vi "Load Display Settings.vi"(8 "error in (no error)":errorcluster, 11 "AF IMAQ Display in":refnum<class "HIJ Vision Display.lvclass">) -> (0 "error out":errorcluster, 3 "AF IMAQ Display out":refnum<class "HIJ Vision Display.lvclass">)   [LabVIEW 2014, in "HIJ Vision Display.lvlib" / "HIJ Vision Display.lvclass"]
uses:
  HIJ Vision Display.lvclass
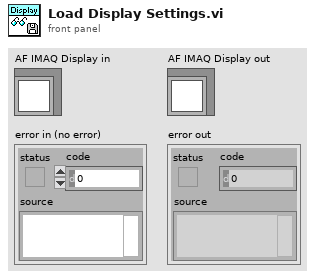
[diagram p1: front panel]
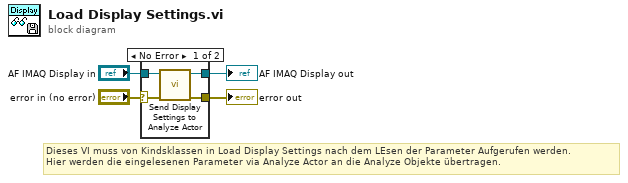
[diagram p0: block diagram]
diagram:
  # "Dieses VI muss von Kindsklassen in Load Display Settings nach dem LEsen der Parameter Aufgerufen werden.\nHier werden die eingelesenen Parameter via Analyze Actor an die Analyze Objekte übertragen."
  n1 = case shown="No Error" "error in (no error)" {
    selector: "error in (no error)" -> [w6 w10]
    tunnel: "AF IMAQ Display in" -> [w8 w9]
    tunnel: [w7 w9] -> w3
    tunnel: [w5 w10] -> w2
    frame No Error {
      n2 = call-dynamic "Send Display Settings to Analyze Actor.vi"("error in (no error)"=w6, "AF IMAQ Display in"=w8) -> ("error out"=w5:errorcluster, "AF IMAQ Display out"=w7:refnum<class "HIJ Vision Display.lvclass">)  [unwired: 8 in]
    }
    frame Error {
    }
  }
  "error out" <- w2
  "AF IMAQ Display out" <- w3
